vi "DMM_GUI.vi"(8 "error in (no error)":errorcluster, 11 "Instrument Reference":u8) -> (0 "error out":errorcluster)   [LabVIEW 2018, in "PXIe-4071.lvclass"]
uses:
  PXIe-4071.lvclass
  DMM Virtual/DMM Virtual.lvclass
panel:
  out "Sub Address":string
  out "Model Number":string
  in  "stop":bool
  # "PXIe-4071 GUI"
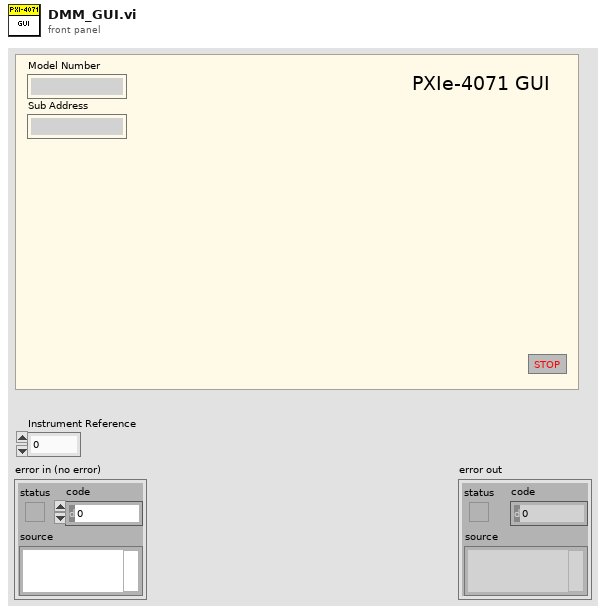
[diagram p1: front panel]
types:
  T1 = typedef "Class Attributes Cluster.ctl" = cluster{"Model Number":string, "Instrument Number":u8, "Rack ID":string, "Inst Mnemonic":string, "Comp Mnemonic":string, "Subsys Mnemonic":string, "IP Address":string, "Sub Address":string, "Firmware Rev":string, "Expected Options":string, "Required Options":string, "Excluded Options":string}
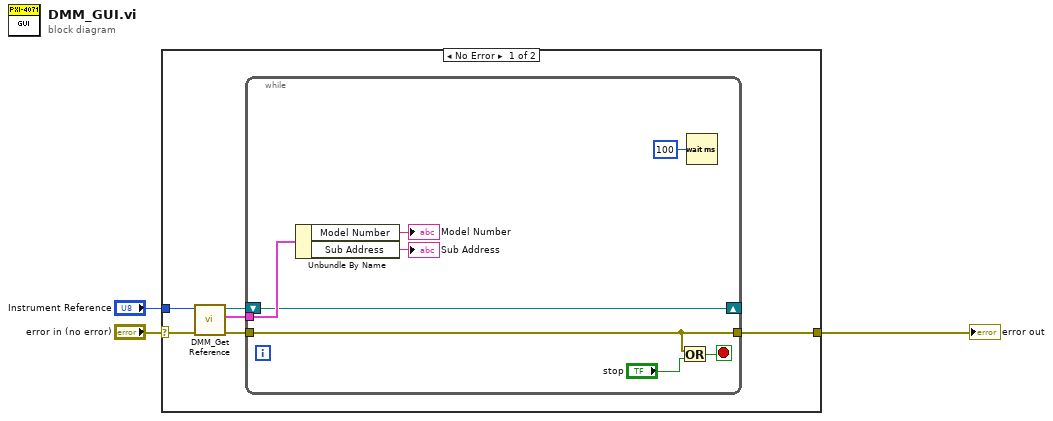
[diagram p0: block diagram]
diagram:
  n1 = case shown="No Error" "error in (no error)" {
    selector: "error in (no error)" -> [w8 w18]
    tunnel: [w9 w18] -> w2
    tunnel: "Instrument Reference" -> [w7 _]
    frame No Error {
      n2 = call "DMM_Get Reference.vi"("error in (no error)"=w8, "Instrument Reference"=w7) -> ("error out"=w6:errorcluster, "Class Attributes"=w4:T1, "DMM Virtual.lvclass"=w5:refnum<class "DMM Virtual.lvclass">)  [unwired: 7 in]
      n3 = while {
        tunnel: w6 -> [w17]
        tunnel: [w17] -> w9
        shift-right: [w10] -> _
        shift-left: w5 -> [w10]
        tunnel: w4 -> [w13]
        stop <- w15 stop-if-true
        n4 = Unbundle By Name(w13) -> ("Model Number"=→"Model Number":string, "Sub Address"=→"Sub Address":string)
        n5 = Or(x=w17, y="stop") -> (x .or. y?=w15:bool)
        n6 = Wait (ms)(milliseconds to wait=u32 100) -> ()  [unwired: 1 out]
      }
    }
    frame Error {
    }
  }
  "error out" <- w2
